vi "ChangeFileExtention.vi"(8 "Error In":errorcluster, 9 "File Extension Separator (.)":string=".", 10 "New extension":string, 11 "File Path":path) -> (0 "Error Out":errorcluster, 1 "Path with new extension":path, 2 "Filename without extension":string, 3 "Path before extension":path, 4 "Old Extension":string, 5 "Name with new extension":string)   [LabVIEW 2019]
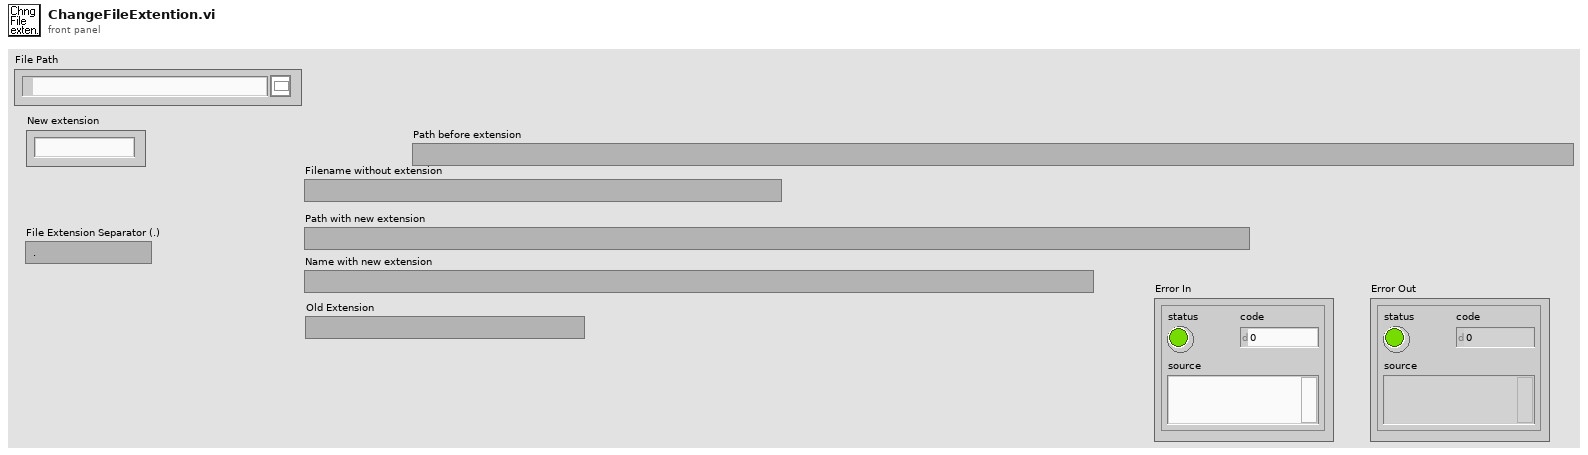
[diagram p1: front panel]
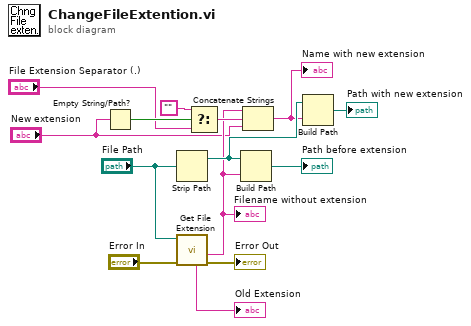
[diagram p0: block diagram]
diagram:
  n1 = Empty String/Path?(string/path="New extension") -> (empty?=w13:bool)
  n2 = Strip Path(path="File Path") -> (stripped path=w8:path)  [unwired: 1 out]
  n3 = call <vilib>:"Get File Extension.vi"("error in (no error)"="Error In", "file"="File Path") -> ("error out"=→"Error Out":errorcluster, "filename without extension"=w6:string, "unmodified file extension"=→"Old Extension":string)  [unwired: 5 in, 2 out]
  "Filename without extension" <- w6
  n4 = Select(t="", s=w13, f="File Extension Separator (.)") -> (s? t:f=w9:string)
  n5 = Build Path(base path=w8, name or relative path=w6) -> (appended path=→"Path before extension":path)
  n6 = Concatenate Strings(w6, w9, "New extension") -> (w5:string)
  "Name with new extension" <- w5
  n7 = Build Path(base path=w8, name or relative path=w5) -> (appended path=→"Path with new extension":path)
